vi "ElevEncActions.vi"(11 "Zero?":bool) -> (3 "ElevEncPos":i32)   [LabVIEW 2018]
uses:
  <vilib>/Rock Robotics/WPI/ThirdParty/Phoenix-LabVIEW/Motor Controller/Get/CTRE_Phoenix_MotorController_GetQuadratureData.vi
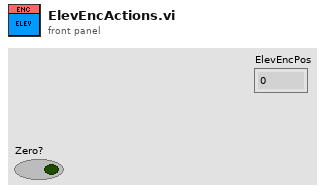
[diagram p1: front panel]
types:
  T1 = typedef "WPI_MotorControlDeviceRef.ctl" = cluster{"DeviceStatus":errorcluster, "Type":T2, "PWM":cluster{"PWM Channel":T3, "DeadBand":T4}, "CAN":cluster{"Device Number":u8, "SetOutput VI Ref":variant, "GetOutput VI Ref":variant, "Enable VI Ref":variant, "Disable VI Ref":variant, "Data":variant}, "Invert":bool, "DIO PWM":cluster{"PWM \"Enable\" Channel":T3, "DIOChannel":T5, "PWM Rate":dbl}}
  T2 = typedef "WPI_MotorControlType.ctl" = enum16{"PWM", "CAN", "DIO PWM"}
  T3 = typedef "FPGA_DIOPWMChannel.ctl" = enum8{"PWM 0", "PWM 1", "PWM 2", "PWM 3", "PWM 4", "PWM 5", "PWM 6", "PWM 7", "PWM 8", "PWM 9", "PWM MXP 0", "PWM MXP 1", "PWM MXP 2", "PWM MXP 3", "PWM MXP 4", "PWM MXP 5", "PWM MXP 6", "PWM MXP 7", "PWM MXP 8", "PWM MXP 9", "Invalid"}
  T4 = typedef "WPI_PWMDeadband.ctl" = cluster{"Name":string, "maxPositivePwm":i32, "minPositivePwm":i32, "centerPwm":i32, "maxNegativePwm":i32, "minNegativePwm":i32, "angularRange":u16}
  T5 = typedef "FPGA_DIOChannel.ctl" = enum8{"DIO 0", "DIO 1", "DIO 2", "DIO 3", "DIO 4", "DIO 5", "DIO 6", "DIO 7", "DIO 8", "DIO 9", "DIO MXP 0", "DIO MXP 1", "DIO MXP 2", "DIO MXP 3", "DIO MXP 4", "DIO MXP 5", "DIO MXP 6", "DIO MXP 7", "DIO MXP 8", "DIO MXP 9", "DIO MXP 10", "DIO MXP 11", "DIO MXP 12", "DIO MXP 13", "DIO MXP 14", "DIO MXP 15", "SPI Port CS1", "SPI Port CS2", "SPI Port CS3", "SPI Port MISO", "SPI Port MOSI", "Invalid"}
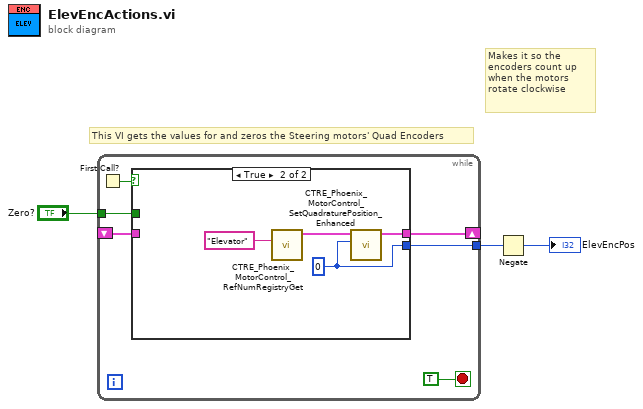
[diagram p0: block diagram]
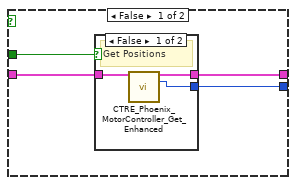
[diagram p2: hidden frame]
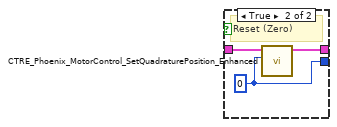
[diagram p3: hidden frame]
diagram:
  # "This VI gets the values for and zeros the Steering motors' Quad Encoders"
  # "Makes it so the encoders count up when the motors rotate clockwise"
  n1 = while {
    shift-right: [w8] -> _
    shift-left: _ -> [w7]
    tunnel: [w9] -> w2
    tunnel: "Zero?" -> [w4]
    stop <- TRUE stop-if-true
    n2 = First Call?() -> (First Call?: T/F=w6:bool)
    n3 = case shown="True" w6 {
      tunnel: w7 -> [w13 _]
      tunnel: [w12 w20] -> w9
      tunnel: [w11 w21] -> w8
      tunnel: w4 -> [w10 _]
      frame False {
        n4 = case shown="False" w10 {
          tunnel: w13 -> [w16 w19]
          tunnel: [w15 w17] -> w12
          tunnel: [w14 w18] -> w11
          frame False {
            # "Get Positions"
            n5 = call-poly <vilib>:"CTRE_Phoenix_MotorController_Get_Enhanced.vi"("PhoenixMotorControlDevRef"=w16) -> ("PhoenixMotorControlDevRef"=w14:T1, "Quadrature Position"=w15:i32)  [unwired: 11 in, 2 out]
          }
          frame True {
            w17 = 0 ("New Position")
            # "Reset (Zero)"
            n6 = call <vilib>:"CTRE_Phoenix_MotorControl_SetQuadraturePosition_Enhanced.vi"("New Position"=w17, "PhoenixMotorControlDevRef"=w19) -> ("PhoenixMotorControlDevRef"=w18:T1)  [unwired: 8 in, 1 out]
          }
        }
      }
      frame True {
        w20 = 0 ("New Sensor Position")
        n7 = call <vilib>:"CTRE_Phoenix_MotorControl_RefNumRegistryGet.vi"("refnum name"="Elevator") -> ("PhoenixMotorControlDevRef"=w22:T1)  [unwired: 9 in, 1 out]
        n8 = call <vilib>:"CTRE_Phoenix_MotorControl_SetQuadraturePosition_Enhanced.vi"("New Position"=w20, "PhoenixMotorControlDevRef"=w22) -> ("PhoenixMotorControlDevRef"=w21:T1)  [unwired: 8 in, 1 out]
      }
    }
  }
  n9 = Negate(x=w2) -> (-x=→"ElevEncPos":i32)
